vi "相机1-保存当前图片为对位时螺丝槽参考图片.vi"(11 "Image In":T4) -> (2 "相机1校准对位时影像坐标":T1 {"坐标"."X" format="%#.3f"}, 3 "Image":T4(plugin-control))   [LabVIEW 2014]
uses:
  Global.vi
  <vilib>/vision/Measure.llb/Edge Polarity.ctl
  <vilib>/vision/Measure.llb/Edge Options.ctl
  <vilib>/vision/Image Controls.llb/IMAQ Image.ctl
  Controls/XYPos.ctl
panel:
  in  "量测项目名称":string[](array[string])=["校准时影像坐标-X", "校准时影像坐标-Y", "校准时影像坐标-角度"]
  in  "Img Path":path=path "E:/771半自动装配系统-2019200427/校准/上相机拍照-螺丝刀原点时-对位完成后拍照螺丝槽.jpg"
  out "Fitted Circle":T3 {"Average SNR (dB)" format="%.2f"; "Average Strength" format="%.2f"; "Roundness (Real-World)" format="%.2f"; "Radius (Real-World)" format="%.2f"; "Center (Real-World)"."Y" format="%.2f"; "Center (Real-World)"."X" format="%.2f"; "Radius (Pixels)" format="%.2f"; "Center (Pixels)"."Y" format="%.2f"; "Center (Pixels)"."X" format="%.2f"}
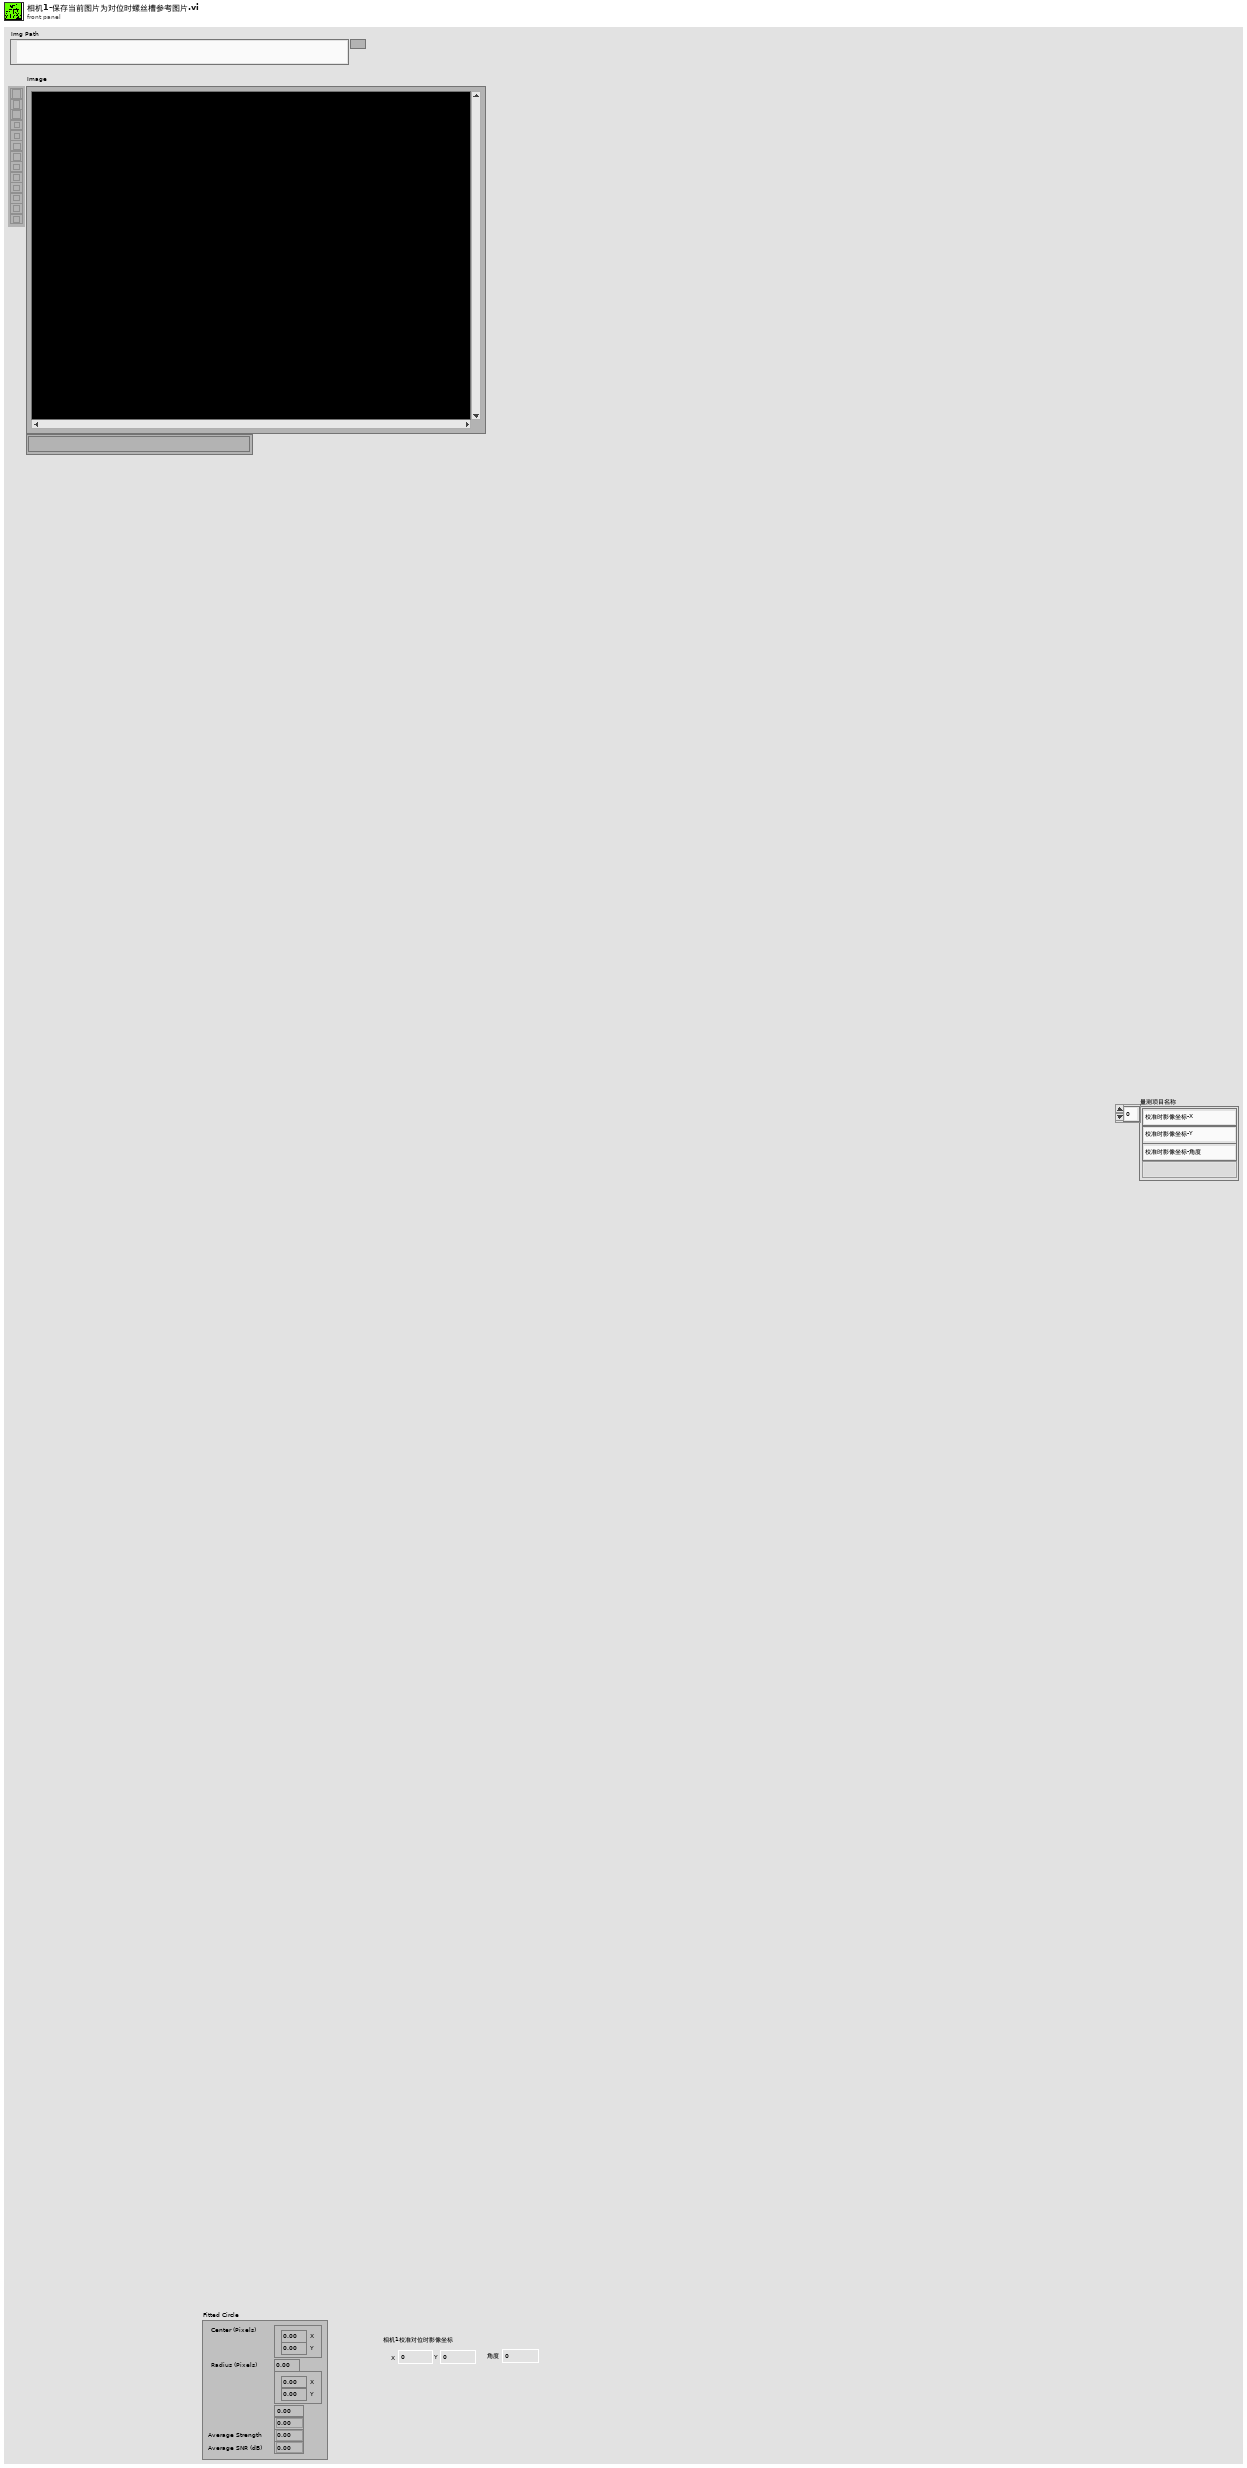
[diagram p1: front panel]
types:
  T1 = typedef "控件-螺丝刀或槽坐标和角度信息.ctl" = cluster{"坐标":T2, "角度":dbl}
  T2 = typedef "XYPos.ctl" = cluster{"X":dbl, "Y":dbl}
  T3 = cluster{"Center (Pixels)":cluster{"X":sgl, "Y":sgl}, "Radius (Pixels)":dbl, "Center (Real-World)":cluster{"X":sgl, "Y":sgl}, "Radius (Real-World)":dbl, "Roundness (Real-World)":dbl, "Average Strength":dbl, "Average SNR (dB)":dbl}
  T4 = typedef "IMAQ Image.ctl" = refnum<image>
  T5 = typedef "Edge Options.ctl" = cluster{"Edge Polarity":T6, "Kernel Size":u32, "Width":u32, "Minimum Edge Strength":sgl, "Interpolation Type":enum32{"Zero Order", "Bilinear", "Quadratic", "Cubic", "Bilinear Fixed"}, "Data Processing Method":enum32{"Average", "Median"}}
  T6 = typedef "Edge Polarity.ctl" = u32
  T7 = cluster{"Search  Direction":u32, "Edge Options":T5, "Show Search Area":bool, "Show Search Lines":bool, "Show Edges Found":bool, "Show Result":bool, "Search Area Color":u32, "Search Lines Color":u32, "Edge Locations Color":u32, "Result Color":u32, "Overlay Group Name":string}
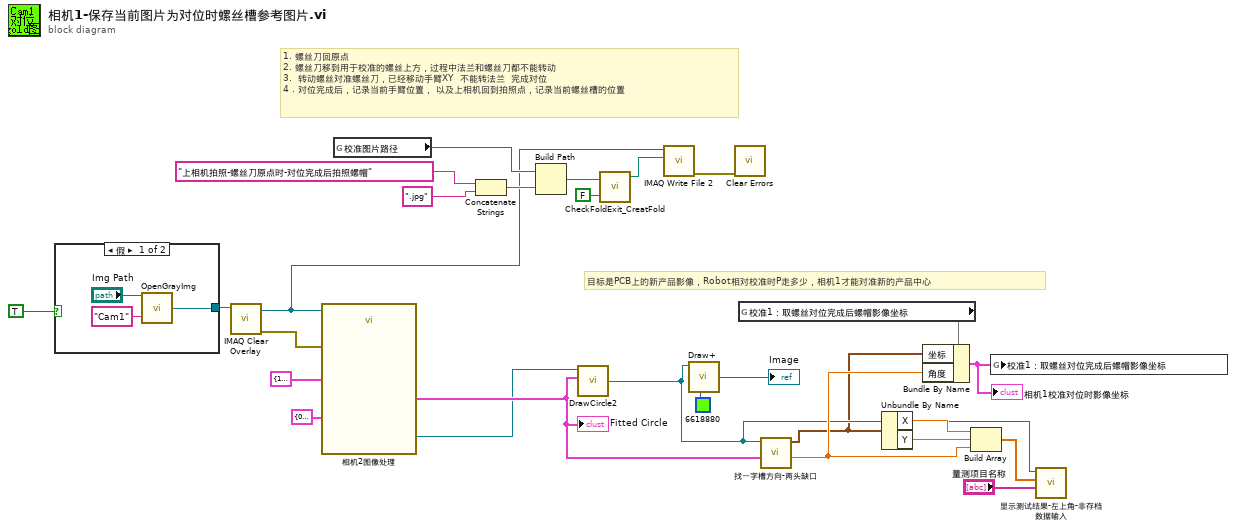
[diagram p0: block diagram]
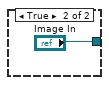
[diagram p2: hidden frame]
diagram:
  # "1. 螺丝刀回原点\n2. 螺丝刀移到用于校准的螺丝上方，过程中法兰和螺丝刀都不能转动\n3.  转动螺丝对准螺丝刀，已经移动手臂XY  不能转法兰  完成对位\n4 . 对位完成后，记录当前手臂位置， 以及上相机回到拍照点，记录当前螺丝槽的位置"
  # "目标是PCB上的新产品影像，Robot相对校准时P走多少，相机1才能对准新的产品中心"
  n1 = case shown="假" TRUE {
    tunnel: [w30 "Image In"] -> w25
    frame False {
      n2 = call "OpenGrayImg.vi"("Image Name"="Cam1", "Img Path"="Img Path") -> ("Image Out"=w30:T4)
    }
    frame True {
    }
  }
  n3 = call "IMAQ Clear Overlay"("Image"=w25) -> ("error out"=w24:errorcluster, "Image Out"=w12:T4)  [unwired: 9 in]
  n4 = call "相机2图像处理"("Image In"=w12, "Options (Find Circular Edge 1)"=T7 {"Search  Direction"=1, "Edge Options"={"Edge Polarity"=0, "Kernel Size"=7, "Width"=3, "Minimum Edge Strength"=30.0, "Interpolation Type"=enum."Bilinear Fixed", "Data Processing Method"=enum."Average"}, "Show Search Area"=FALSE, "Show Search Lines"=FALSE, "Show Edges Found"=FALSE, "Show Result"=TRUE, "Search Area Color"=65280, "Search Lines Color"=255, "Edge Locations Color"=16776960, "Result Color"=16711680, "Overlay Group Name"=""}, "Options (定位圆)"=T7 {"Search  Direction"=0, "Edge Options"={"Edge Polarity"=2, "Kernel Size"=5, "Width"=5, "Minimum Edge Strength"=50.0, "Interpolation Type"=enum."Bilinear Fixed", "Data Processing Method"=enum."Average"}, "Show Search Area"=FALSE, "Show Search Lines"=FALSE, "Show Edges Found"=TRUE, "Show Result"=FALSE, "Search Area Color"=65280, "Search Lines Color"=255, "Edge Locations Color"=16776960, "Result Color"=16711680, "Overlay Group Name"=""}, "error in"=w24) -> ("Image Out"=w4:T4, "Fitted Circle (Find Circular Edge 1)"=w5:T3)  [unwired: 21 in, 1 out]
  "Fitted Circle" <- w5
  n5 = global read "Global.vi" "校准图片路径"() -> (w20:path)
  n6 = Concatenate Strings("上相机拍照-螺丝刀原点时-对位完成后拍照螺帽" ("time format string (%c)"), ".jpg" ("字符串")) -> (w19:string)
  n7 = Build Path(base path=w20, name or relative path=w19) -> (appended path=w15:path)
  n8 = call "DrawCircle2.vi"("Fitted Circle (左圆)"=w5, "Img in"=w4) -> ("Img out"=w3:T4)  [unwired: 2 in]
  n9 = call "CheckFoldExit_CreatFold.vi"("path in"=w15, "FoldOrFile¡H"=FALSE) -> ("File out"=w13:path)  [unwired: 2 out]
  n10 = call-poly "IMAQ Write File 2"("File Path"=w13, "Image"=w12) -> ("error out"=w18:errorcluster)  [unwired: 8 in, 1 out]
  n11 = call "Draw+.vi"("Color"=u32 6618880, "Image In"=w3) -> ("Image Out"=→"Image":T4)  [unwired: 4 in]
  n12 = call <vilib>:"Clear Errors.vi"("error in (no error)"=w18) -> ()  [unwired: 5 in, 2 out]
  n13 = global read "Global.vi" "校准1：取螺丝对位完成后螺帽影像坐标"() -> (w23)
  n14 = call "找一字槽方向-两头缺口.vi"("Fitted Circle"=w5, "Img in"=w3) -> ("一字槽角度"=w7:dbl, "一字槽中心"=w1:cluster{"X":sgl, "Y":sgl})  [unwired: 7 in, 1 out]
  n15 = Unbundle By Name(w1) -> ("X"=w9:sgl, "Y"=w8:sgl)
  n16 = Bundle By Name(cluster=w23, "坐标"=w1, "角度"=w7) -> (w22:cluster{})
  "相机1校准对位时影像坐标" <- w22
  n17 = Build Array(w9, w8, w7) -> (w6:dbl[])
  n18 = global write "Global.vi" "校准1：取螺丝对位完成后螺帽影像坐标"(w22) -> ()
  n19 = call "显示测试结果-左上角-非存档数据输入.vi"("量测项目名称"="量测项目名称", "显示数据"=w6, "Img输入"=w3) -> ()  [unwired: 8 in, 1 out]
